vi "Trim Library From Name.vi"(1 "Name in":string) -> (0 "Name out":string)   [LabVIEW 2018, in "Templates.lvlib"]
uses:
  Templates.lvlib
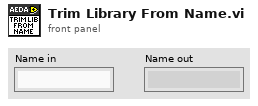
[diagram p1: front panel]
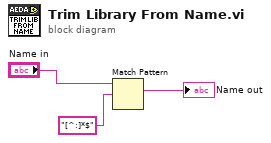
[diagram p0: block diagram]
diagram:
  n1 = Match Pattern(string="Name in", regular expression="[^:]*$") -> (match substring=→"Name out":string)  [unwired: 1 in, 3 out]
